vi "BlinkLight.vi"() -> (0 "Blinked":bool)   [LabVIEW 2019]
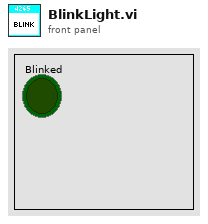
[diagram p1: front panel]
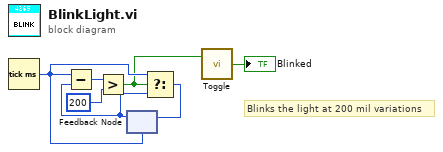
[diagram p0: block diagram]
diagram:
  # "Blinks the light at 200 mil variations"
  n1 = Tick Count (ms)() -> (millisecond timer value=w6:u32)
  n2 = feedback #1(w6) -> (w5:u32)
  n3 = Subtract(x=w6, y=w5) -> (x-y=w3:u32)
  n4 = Greater?(x=w3, y=u32 200) -> (0:w4:bool)
  n5 = Select(t=w6, s=w4, f=w5) -> (s? t:f=w7:u32)
  n6 = feedback-in #1(w7) -> ()
  n7 = call "Toggle.vi"("Trigger"=w4) -> ("New State"=→"Blinked":bool)  [unwired: 1 in]
